vi "Start Test.vi"(8 "error in (no error)":errorcluster, 10 "Tests":string[](array[string]), 11 "Result Model In":refnum<class "Result Model.lvclass">) -> (0 "error out":errorcluster, 3 "Result Model Out":refnum<class "Result Model.lvclass">)   [LabVIEW 2020, in "Result Model.lvclass"]
uses:
  Result Model.lvclass
  Result Model.lvclass/Result Model.ctl
  Core/Result/Status.ctl
  Core/Result/Result.lvlib
  0a8f46ae-0ef9-419d-aab8-e3e68aadb659.vi
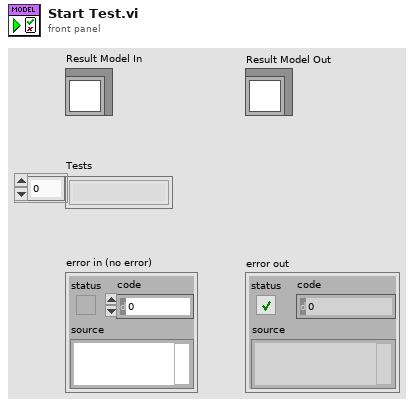
[diagram p1: front panel]
types:
  T1 = typedef "Result.lvlib/Status.ctl" = enum16{"", "Passed", "Failed", "Error", "Skipped", "Setup Error", "Broken", "Teardown Error"}
  T2 = typedef "Result.lvlib/Type.ctl" = enum16{"Test Case", "Test Suite", "Test Run", "Pass", "Fail", "Skip", "Pass if", "Fail if", "Pass if Error", "Fail if Error", "Pass if Equal", "Fail if Equal"}
  T3 = map{string, cluster{"Result Type":T2, "Status":T1, "Description":string, "Data":cluster{"Expected":variant, "Actual":variant, "Delta":variant}}[]}
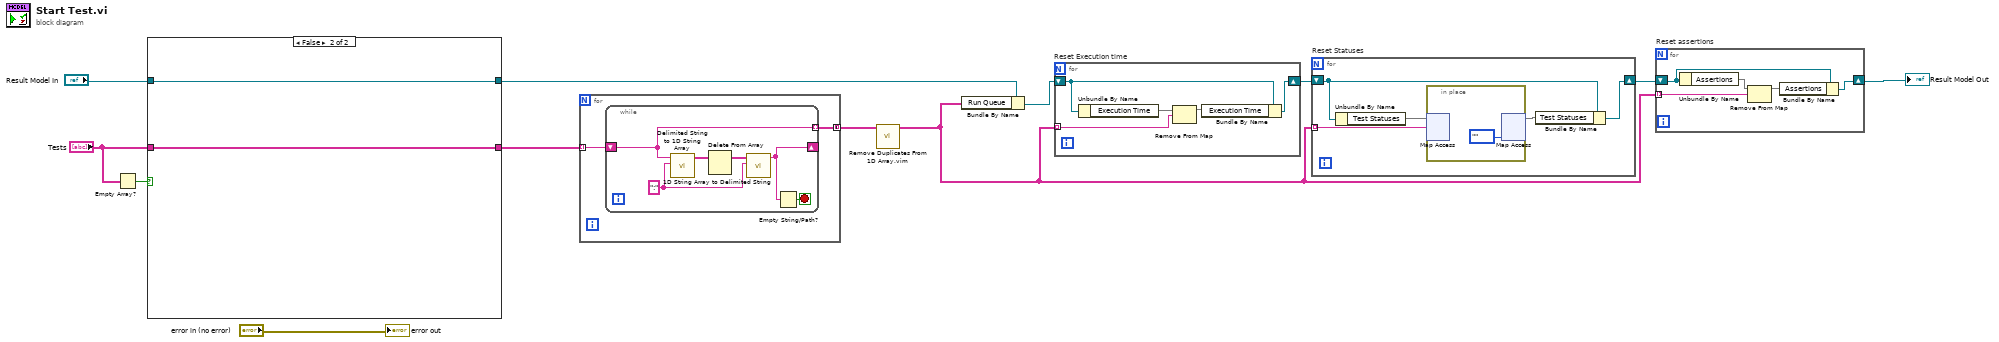
[diagram p0: block diagram]
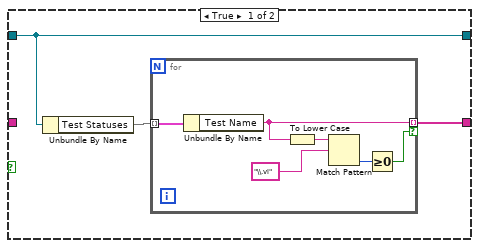
[diagram p2: hidden frame]
diagram:
  n1 = Empty Array?(array="Tests") -> (empty?=w11:bool)
  n2 = case shown="False" w11 {
    tunnel: "Result Model In" -> [w14 w23]
    tunnel: [w14 w23] -> w8
    tunnel: "Tests" -> [_ w22]
    tunnel: [w13 w22] -> w9
    frame True {
      n3 = Unbundle By Name(w14) -> ("Test Statuses"=w15:map{string, T1})
      n4 = for {
        tunnel: w15 -> [w21] mode=indexing
        tunnel: [w17] -> w13 mode=indexing if=w16
        n5 = Unbundle By Name(w21) -> ("Test Name"=w17:string)
        n6 = To Lower Case(string=w17) -> (all lower case string=w18:string)
        n7 = Match Pattern(string=w18, regular expression="\\.vi") -> (offset past match=w19:i32)  [unwired: 1 in, 3 out]
        n8 = Greater Or Equal To 0?(x=w19) -> (x >= 0?=w16:bool)
      }
    }
    frame False {
    }
  }
  n9 = for {
    tunnel: w9 -> [w25] mode=indexing
    tunnel: [w24] -> w2 mode=concatenating
    n10 = while {
      shift-right: [w27] -> _
      shift-left: w25 -> [w26]
      tunnel: [w26] -> w24 mode=indexing
      stop <- w28 stop-if-true
      w30 = ":" ("delimiter")
      n11 = call <vilib>:"Delimited String to 1D String Array.vi"("delimiter"=w30, "delimited string"=w26) -> ("string array"=w31:string[])  [unwired: 9 in]
      n12 = Delete From Array(array=w31) -> (array with subset deleted=w29:string[])  [unwired: 2 in, 1 out]
      n13 = call <vilib>:"1D String Array to Delimited String.vi"("delimiter"=w30, "string array"=w29) -> ("delimited string"=w27:string)  [unwired: 9 in]
      n14 = Empty String/Path?(string/path=w27) -> (empty?=w28:bool)
    }
  }
  n15 = call "Remove Duplicates From 1D Array.vim"("array"=w2) -> ("array with duplicates removed"=w1:string[])  [unwired: 10 in]
  n16 = Bundle By Name(cluster=w8, "Run Queue"=w1) -> (w4:refnum<class "Result Model.lvclass">)
  n17 = for "Reset Execution time" {
    tunnel: w1 -> [w36] mode=indexing
    shift-right: [w32] -> w5
    shift-left: w4 -> [w33]
    n18 = Unbundle By Name(w33) -> ("Execution Time"=w35:map{string, dbl})
    n19 = Remove From Map(10:w36, 11:w35) -> (3:w34:map{string, dbl})  [unwired: 2 out]
    n20 = Bundle By Name(cluster=w33, "Execution Time"=w34) -> (w32:refnum<class "Result Model.lvclass">)
  }
  n21 = for "Reset Statuses" {
    tunnel: w1 -> [w41] mode=indexing
    shift-right: [w37] -> w6
    shift-left: w5 -> [w38]
    n22 = Unbundle By Name(w38) -> ("Test Statuses"=w40:map{string, T1})
    n23 = in-place {
      n24 = in-place-map #1(w40, w41) -> ()  [unwired: 1 in, 2 out]
      n25 = in-place-map #1(Status."" ("value")) -> (w39:map{string, T1})  [unwired: 1 in, 2 out]
    }
    n26 = Bundle By Name(cluster=w38, "Test Statuses"=w39) -> (w37:refnum<class "Result Model.lvclass">)
  }
  n27 = for "Reset assertions" {
    tunnel: w1 -> [w47] mode=indexing
    shift-right: [w43] -> w3
    shift-left: w6 -> [w44]
    n28 = Unbundle By Name(w44) -> ("Assertions"=w46:T3)
    n29 = Remove From Map(10:w47, 11:w46) -> (3:w45:T3)  [unwired: 2 out]
    n30 = Bundle By Name(cluster=w44, "Assertions"=w45) -> (w43:refnum<class "Result Model.lvclass">)
  }
  "Result Model Out" <- w3
  "error out" <- "error in (no error)"
